vi "Get Channel Service.vi"(8 "error in (no error)":errorcluster, 11 "Vecto in":refnum<class "Vecto.lvclass">) -> (0 "error out":errorcluster, 2 "ChannelService":refnum<class "ChannelService.lvclass">, 3 "Vecto out":refnum<class "Vecto.lvclass">)   [LabVIEW 2020, in "Vecto.lvlib" / "Vecto.lvclass"]
uses:
  Vecto.lvclass
  ChannelService/ChannelService.lvclass
  Vecto.lvclass/Vecto.ctl
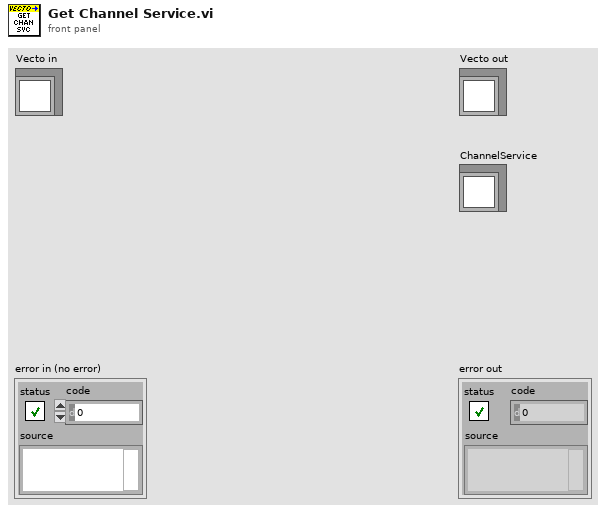
[diagram p1: front panel]
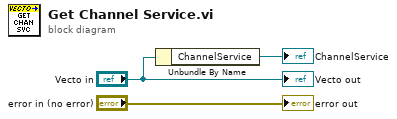
[diagram p0: block diagram]
diagram:
  n1 = Unbundle By Name("Vecto in") -> ("ChannelService"=→"ChannelService":refnum<class "ChannelService.lvclass">)
  "error out" <- "error in (no error)"
  "Vecto out" <- "Vecto in"
